vi "Distance IR Bricklet Test.vi"() -> ()   [LabVIEW 2011]
uses:
  Classes/Device/Type Definitions/Callback Option.ctl
  Classes/IP Connection/IP Connection.lvclass
  Classes/Device/Device.lvclass
  Classes/Distance IR Bricklet/Distance IR Bricklet.lvclass
panel:
  out "appended array":bool[](array[boolean])
  out "x-y":u32
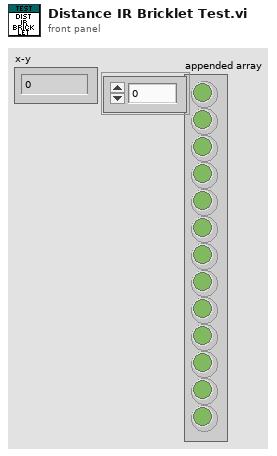
[diagram p1: front panel]
types:
  T1 = typedef "Tinkerforge.lvlib/Device.lvclass/Callback Option.ctl" = enum8{"CB off", "outside range", "inside range", "smaller", "greater"}
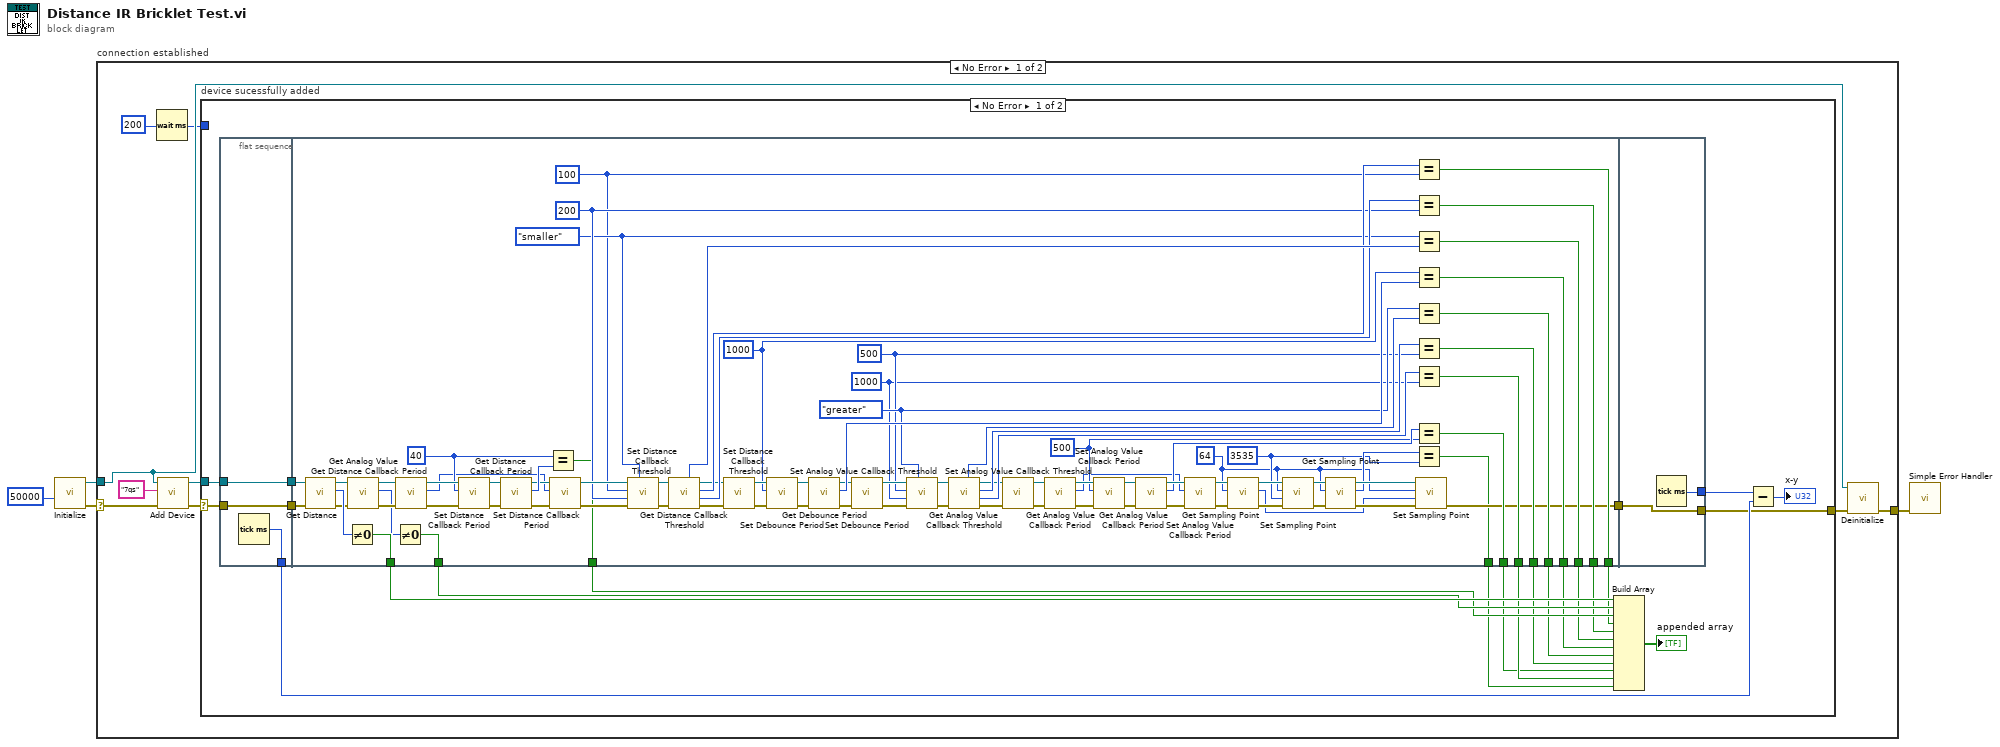
[diagram p0: block diagram]
diagram:
  n1 = call "Initialize.vi"("Timeout (2500ms)"=50000) -> ("error out"=w2:errorcluster, "IP Connection out"=w4:refnum<class "IP Connection.lvclass">)  [unwired: 9 in]
  n2 = case "connection established" shown="No Error" w2 {
    selector: w2 -> [w9 w127]
    tunnel: w4 -> [w13 _]
    tunnel: [w5 w127] -> w3
    frame No Error {
      n3 = Wait (ms)(milliseconds to wait=u32 200) -> (millisecond timer value=w6:u32)
      n4 = call "Add Device.vi"("Error In"=w9, "Device UID"="7qs", "IP Connection"=w13) -> ("Error Out"=w8:errorcluster, "Distance IR Bricklet"=w10:refnum<class "Distance IR Bricklet.lvclass">)  [unwired: 7 in]
      n5 = case "device sucessfully added" shown="No Error" w8 {
        selector: w8 -> [w35 w126]
        tunnel: [w15 w126] -> w11
        tunnel: w10 -> [w34 _]
        tunnel: w6 -> [_ _]
        frame No Error {
          n6 = flat-sequence {
            tunnel: w34 -> [w37]
            tunnel: w35 -> [w38]
            tunnel: [w38] -> w32
            tunnel: [w37] -> w31
            tunnel: [w36] -> w29
            tunnel: [w44] -> w33
            tunnel: w32 -> [w123]
            tunnel: w31 -> [w122]
            tunnel: [w68] -> w27
            tunnel: [w67] -> w26
            tunnel: [w66] -> w25
            tunnel: [w65] -> w24
            tunnel: [w64] -> w23
            tunnel: [w63] -> w22
            tunnel: [w62] -> w21
            tunnel: [w61] -> w20
            tunnel: [w60] -> w19
            tunnel: [w59] -> w18
            tunnel: [w58] -> w17
            tunnel: [w41] -> w14
            tunnel: [w125] -> w15
            tunnel: w33 -> [w125]
            tunnel: [w124] -> w30
            frame #0 {
              n7 = Tick Count (ms)() -> (millisecond timer value=w36:u32)
            }
            frame #1 {
              w40 = u8 64 ("position")
              w42 = u16 3535 ("emissivity")
              w70 = u32 500 ("period (0: off)")
              w82 = i16 1000 ("max")
              w84 = i16 500 ("min")
              w87 = Callback_Option."greater" ("Callback Option (off)")
              w97 = u32 1000 ("debounce (100)")
              w105 = i16 200 ("max")
              w90 = i16 100 ("min")
              w91 = Callback_Option."smaller" ("Callback Option (off)")
              w116 = u32 40
              n8 = call "Get Distance.vi"("error in (no error)"=w123, "Distance IR Bricklet in"=w122) -> ("error out"=w57:errorcluster, "Distance"=w115:u16, "Distance IR Bricklet out"=w56:refnum<class "Distance IR Bricklet.lvclass">)  [unwired: 7 in]
              n9 = Not Equal To 0?(x=w115) -> (x != 0?=w68:bool)
              n10 = call "Get Analog Value.vi"("error in (no error)"=w57, "Distance IR Bricklet in"=w56) -> ("error out"=w55:errorcluster, "Analog Value"=w54:u16, "Distance IR Bricklet out"=w53:refnum<class "Distance IR Bricklet.lvclass">)  [unwired: 7 in]
              n11 = Not Equal To 0?(x=w54) -> (x != 0?=w67:bool)
              n12 = call "Get Distance Callback Period.vi"("error in (no error)"=w55, "Distance IR Bricklet in"=w53) -> ("error out"=w121:errorcluster, "period"=w112:u32, "Distance IR Bricklet out"=w118:refnum<class "Distance IR Bricklet.lvclass">)  [unwired: 7 in]
              n13 = call "Set Distance Callback Period.vi"("error in (no error)"=w121, "period (0: off)"=w116, "Distance IR Bricklet in"=w118) -> ("error out"=w120:errorcluster, "Distance IR Bricklet out"=w119:refnum<class "Distance IR Bricklet.lvclass">)  [unwired: 7 in]
              n14 = call "Get Distance Callback Period.vi"("error in (no error)"=w120, "Distance IR Bricklet in"=w119) -> ("error out"=w114:errorcluster, "period"=w117:u32, "Distance IR Bricklet out"=w113:refnum<class "Distance IR Bricklet.lvclass">)  [unwired: 7 in]
              n15 = Equal?(x=w116, y=w117) -> (x = y?=w66:bool)
              n16 = call "Set Distance Callback Period.vi"("error in (no error)"=w114, "period (0: off)"=w112, "Distance IR Bricklet in"=w113) -> ("error out"=w111:errorcluster, "Distance IR Bricklet out"=w109:refnum<class "Distance IR Bricklet.lvclass">)  [unwired: 7 in]
              n17 = call "Set Distance Callback Threshold.vi"("Callback Option (off)"=w91, "error in (no error)"=w111, "max"=w105, "min"=w90, "Distance IR Bricklet in"=w109) -> ("error out"=w110:errorcluster, "Distance IR Bricklet out"=w104:refnum<class "Distance IR Bricklet.lvclass">)  [unwired: 5 in]
              n18 = call "Get Distance Callback Threshold.vi"("error in (no error)"=w110, "Distance IR Bricklet in"=w104) -> ("error out"=w103:errorcluster, "max"=w106:i16, "min"=w107:i16, "Distance IR Bricklet out"=w102:refnum<class "Distance IR Bricklet.lvclass">, "Callback Option"=w108:T1)  [unwired: 5 in]
              n19 = call "Set Distance Callback Threshold.vi"("error in (no error)"=w103, "Distance IR Bricklet in"=w102) -> ("error out"=w101:errorcluster, "Distance IR Bricklet out"=w100:refnum<class "Distance IR Bricklet.lvclass">)  [unwired: 8 in]
              n20 = call "Set Debounce Period.vi"("error in (no error)"=w101, "debounce (100)"=w97, "Distance IR Bricklet in"=w100) -> ("error out"=w98:errorcluster, "Distance IR Bricklet out"=w99:refnum<class "Distance IR Bricklet.lvclass">)  [unwired: 7 in]
              n21 = call "Get Debounce Period.vi"("error in (no error)"=w98, "Distance IR Bricklet in"=w99) -> ("error out"=w95:errorcluster, "debounce"=w96:u32, "Distance IR Bricklet out"=w94:refnum<class "Distance IR Bricklet.lvclass">)  [unwired: 7 in]
              n22 = call "Set Debounce Period.vi"("error in (no error)"=w95, "Distance IR Bricklet in"=w94) -> ("error out"=w93:errorcluster, "Distance IR Bricklet out"=w92:refnum<class "Distance IR Bricklet.lvclass">)  [unwired: 8 in]
              n23 = call "Set Analog Value Callback Threshold.vi"("Callback Option (off)"=w87, "error in (no error)"=w93, "max"=w82, "min"=w84, "Distance IR Bricklet in"=w92) -> ("error out"=w89:errorcluster, "Distance IR Bricklet out"=w88:refnum<class "Distance IR Bricklet.lvclass">)  [unwired: 5 in]
              n24 = call "Get Analog Value Callback Threshold.vi"("error in (no error)"=w89, "Distance IR Bricklet in"=w88) -> ("error out"=w81:errorcluster, "max"=w83:i16, "min"=w85:i16, "Distance IR Bricklet out"=w80:refnum<class "Distance IR Bricklet.lvclass">, "Callback Option"=w86:T1)  [unwired: 5 in]
              n25 = call "Set Analog Value Callback Threshold.vi"("error in (no error)"=w81, "Distance IR Bricklet in"=w80) -> ("error out"=w79:errorcluster, "Distance IR Bricklet out"=w78:refnum<class "Distance IR Bricklet.lvclass">)  [unwired: 8 in]
              n26 = call "Get Analog Value Callback Period.vi"("error in (no error)"=w79, "Distance IR Bricklet in"=w78) -> ("error out"=w77:errorcluster, "period"=w69:u32, "Distance IR Bricklet out"=w76:refnum<class "Distance IR Bricklet.lvclass">)  [unwired: 7 in]
              n27 = call "Set Analog Value Callback Period.vi"("error in (no error)"=w77, "period (0: off)"=w70, "Distance IR Bricklet in"=w76) -> ("error out"=w74:errorcluster, "Distance IR Bricklet out"=w73:refnum<class "Distance IR Bricklet.lvclass">)  [unwired: 7 in]
              n28 = call "Get Analog Value Callback Period.vi"("error in (no error)"=w74, "Distance IR Bricklet in"=w73) -> ("error out"=w72:errorcluster, "period"=w71:u32, "Distance IR Bricklet out"=w75:refnum<class "Distance IR Bricklet.lvclass">)  [unwired: 7 in]
              n29 = call "Set Analog Value Callback Period.vi"("error in (no error)"=w72, "period (0: off)"=w69, "Distance IR Bricklet in"=w75) -> ("error out"=w52:errorcluster, "Distance IR Bricklet out"=w51:refnum<class "Distance IR Bricklet.lvclass">)  [unwired: 7 in]
              n30 = call "Get Sampling Point.vi"("error in (no error)"=w52, "position"=w40, "Distance IR Bricklet in"=w51) -> ("error out"=w50:errorcluster, "distance"=w39:u16, "Distance IR Bricklet out"=w49:refnum<class "Distance IR Bricklet.lvclass">)  [unwired: 6 in]
              n31 = call "Set Sampling Point.vi"("error in (no error)"=w50, "distance"=w42, "position"=w40, "Distance IR Bricklet in"=w49) -> ("error out"=w47:errorcluster, "Distance IR Bricklet out"=w46:refnum<class "Distance IR Bricklet.lvclass">)  [unwired: 6 in]
              n32 = call "Get Sampling Point.vi"("error in (no error)"=w47, "position"=w40, "Distance IR Bricklet in"=w46) -> ("error out"=w48:errorcluster, "distance"=w43:u16, "Distance IR Bricklet out"=w45:refnum<class "Distance IR Bricklet.lvclass">)  [unwired: 6 in]
              n33 = Equal?(x=w107, y=w90) -> (x = y?=w65:bool)
              n34 = Equal?(x=w106, y=w105) -> (x = y?=w64:bool)
              n35 = Equal?(x=w91, y=w108) -> (x = y?=w63:bool)
              n36 = Equal?(x=w97, y=w96) -> (x = y?=w62:bool)
              n37 = Equal?(x=w87, y=w86) -> (x = y?=w61:bool)
              n38 = Equal?(x=w85, y=w84) -> (x = y?=w60:bool)
              n39 = Equal?(x=w83, y=w82) -> (x = y?=w59:bool)
              n40 = Equal?(x=w71, y=w70) -> (x = y?=w58:bool)
              n41 = Equal?(x=w43, y=w42) -> (x = y?=w41:bool)
              n42 = call "Set Sampling Point.vi"("error in (no error)"=w48, "distance"=w39, "position"=w40, "Distance IR Bricklet in"=w45) -> ("error out"=w44:errorcluster)  [unwired: 6 in, 1 out]
            }
            frame #2 {
              n43 = Tick Count (ms)() -> (millisecond timer value=w124:u32)
            }
          }
          n44 = Build Array(w27, w26, w25, w24, w23, w22, w21, w20, w19, w17, w18, w14) -> (→"appended array":bool[])
          n45 = Subtract(x=w30, y=w29) -> (x-y=→"x-y":u32)
        }
        frame Error {
        }
      }
      n46 = call "Deinitialize.vi"("error in (no error)"=w11, "IP Connection in"=w13) -> ("error out"=w5:errorcluster)  [unwired: 9 in]
    }
    frame Error {
    }
  }
  n47 = call <vilib>:"Simple Error Handler.vi"("error in (no error)"=w3) -> ()  [unwired: 4 in, 5 out]
